vi "XIPIN_Processor_System_Reset_5_0.vi"   [LabVIEW 2017]
doc: "Processor Reset System\n------------------------------------\n<b>Need License</b> : No"
uses:
  <vilib>/rvi/XilinxIP/XIPIN_XNode/niFpgaXIPIN.xnode
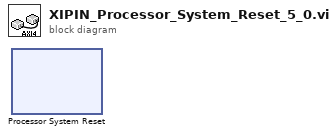
[diagram p0: block diagram]
diagram:
  n1 = xnode ("Processor System Reset")() -> ()
